vi "Simple Error Handler.vi"(6 "Dialog Type":T2, 7 "Window Title":string, 8 "Error In":errorcluster) -> (0 "Error Out":errorcluster, 3 "User Action":T1)   [LabVIEW 2016, in "Stream Error.lvlib"]
doc: "--\nCopyright © 2017 Composed SystemsI All rights reserved.\n\nAuthor: Jon McBee <jon.mcbee@composed.io>\n\nThis library is provided \"AS IS\" ,WITHOUT WARRANTIES OR\nCONDITIONS OF ANY KIND, either express or implied.\n\nComposed Systems -- composed.io\n\nStream 0.0.1.1\nJon McBee - Composed Systems\nCopyright (c) 2017, Composed Systems"
uses:
  <userlib>/Composed Systems/Stream/Error/Stream Error.lvlib
  <userlib>/Composed Systems/Stream/Error/Classes/Error Interface/Dialog Types.ctl
  <userlib>/Composed Systems/Stream/Error/Classes/Error Interface/User Actions.ctl
  <userlib>/Composed Systems/Stream/Error/Classes/Error Interface/Error UID.ctl
  <userlib>/Composed Systems/Stream/Error/Classes/Error Interface/Error Interface.lvclass
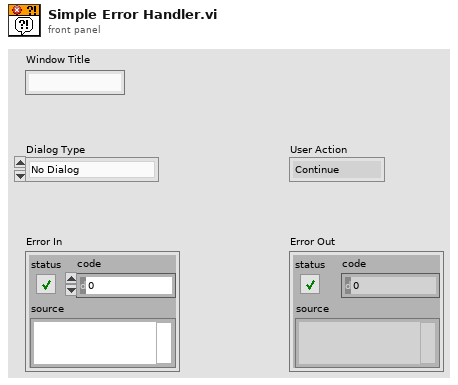
[diagram p1: front panel]
types:
  T1 = typedef "Stream Error.lvlib/Error Interface.lvclass/User Actions.ctl" = enum16{"Continue", "Stop", "Abort"}
  T2 = typedef "Stream Error.lvlib/Error Interface.lvclass/Dialog Types.ctl" = enum16{"No Dialog", "Continue Dialog", "Stop Dialog", "Abort Dialog"}
  T3 = typedef "Stream Error.lvlib/Error Interface.lvclass/Error UID.ctl" = u16
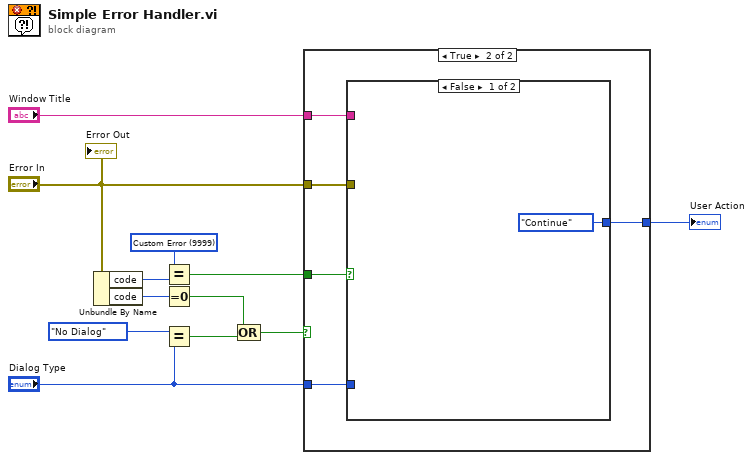
[diagram p0: block diagram]
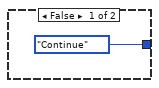
[diagram p2: hidden frame]
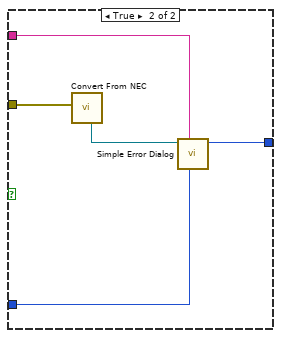
[diagram p3: hidden frame]
diagram:
  w9 = T3 9999 items=["Custom Error"=9999] ("Custom Error Codes")
  n1 = Unbundle By Name("Error In") -> ("code"=w10:i32, "code"=w7:i32)
  n2 = Equal?(x=w9, y=w10) -> (x = y?=w8:bool)
  n3 = Equal To 0?(x=w7) -> (x = 0?=w5:bool)
  n4 = Equal?(x=Dialog_Types."No Dialog" ("Dialog Type"), y="Dialog Type") -> (x = y?=w4:bool)
  n5 = Compound Arithmetic op=OR(w5, w4) -> (w3:bool)
  n6 = case shown="True" w3 {
    tunnel: "Error In" -> [_ w17]
    tunnel: "Window Title" -> [_ w16]
    tunnel: w8 -> [_ w18]
    tunnel: "Dialog Type" -> [_ w15]
    tunnel: [User_Actions."Continue" ("User Action") w14] -> w1
    frame False {
    }
    frame True {
      n7 = case shown="False" w18 {
        tunnel: w17 -> [_ w22]
        tunnel: w16 -> [_ w23]
        tunnel: w15 -> [_ w24]
        tunnel: [User_Actions."Continue" ("User Action") w20] -> w14
        frame False {
        }
        frame True {
          n8 = call <userlib>:"Convert From NEC.vi"("error in (no error)"=w22) -> ("Error Interface out"=w21:refnum<class "Error Interface.lvclass">)  [unwired: 9 in, 1 out]
          n9 = call-dynamic "Simple Error Dialog.vi"("Dialog Type"=w24, "Window Title"=w23, "Error Interface in"=w21) -> ("User Action"=w20:T1)  [unwired: 8 in]
        }
      }
    }
  }
  "User Action" <- w1
  "Error Out" <- "Error In"
